vi "Get Iteration.vi"(11 "Framework in":refnum<class "Framework.lvclass">) -> (2 "iteration":u64, 3 "Framework out":refnum<class "Framework.lvclass">)   [LabVIEW 2017, in "DSF Core.lvlib" / "Framework.lvclass"]
uses:
  Framework.lvclass
  Framework.lvclass/Framework.ctl
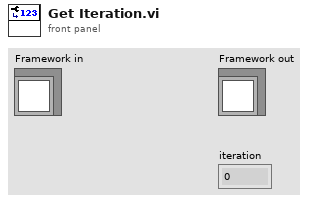
[diagram p1: front panel]
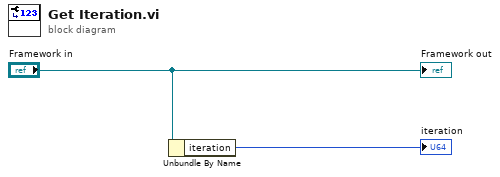
[diagram p0: block diagram]
diagram:
  n1 = Unbundle By Name("Framework in") -> ("iteration"=→"iteration":u64)
  "Framework out" <- "Framework in"
